vi "Stylus.vi"(9 "Position":T1 {"z (mm)" format="%.1f"; "y (mm)" format="%.1f"; "x (mm)" format="%.1f"}, 10 "Radius":dbl=0.4000000059604645) -> (1 "3D Picture":refnum<vi>(3d-picture), 3 "Scene Object Out":refnum<vi>)   [LabVIEW 2023]
uses:
  <vilib>/picture/3D Picture Control/Object/Create Object (name).vi
  <vilib>/picture/3D Picture Control/Object/Add Object (no reference).vi
  <vilib>/picture/3D Picture Control/NI_3D Picture Control.lvlib
panel:
  out "error out":errorcluster
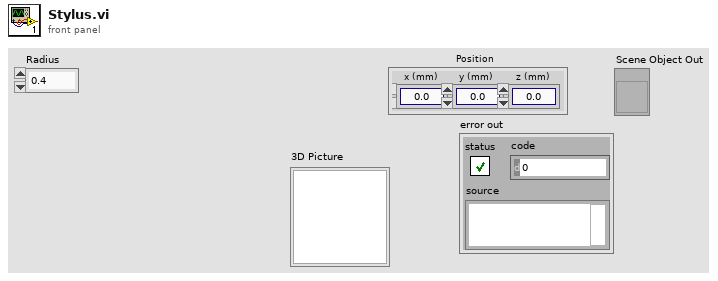
[diagram p1: front panel]
types:
  T1 = cluster{"x (mm)":dbl, "y (mm)":dbl, "z (mm)":dbl}
  T2 = cluster{"Red":sgl, "Green":sgl, "Blue":sgl, "Alpha":sgl}
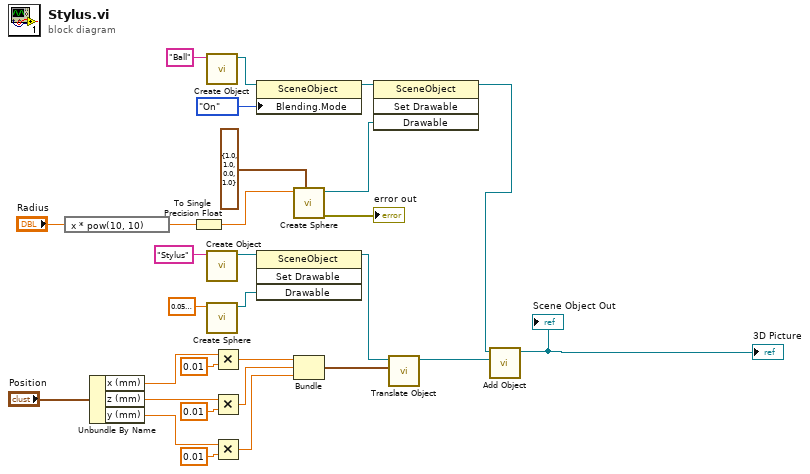
[diagram p0: block diagram]
diagram:
  n1 = expression code="x * pow(10, 10)"("Radius") -> (w9:dbl)
  n2 = Unbundle By Name("Position") -> ("x (mm)"=w19:dbl, "z (mm)"=w18:dbl, "y (mm)"=w17:dbl)
  n3 = To Single Precision Float(number=w9) -> (single precision float=w8:sgl)
  n4 = call-poly <vilib>:"Create Object.vi"("Name"="Ball") -> ("Scene:New Object"=w6:refnum<vi>)  [unwired: 9 in, 1 out]
  n5 = call-poly <vilib>:"Create Object.vi"("Name"="Stylus") -> ("Scene:New Object"=w27:refnum<vi>)  [unwired: 9 in, 1 out]
  n6 = call <vilib>:"Create Sphere.vi"("Radius"=sgl 0.05) -> ("New Sphere Refnum"=w26:refnum<vi>)  [unwired: 9 in, 1 out]
  n7 = Multiply(x=w19, y=0.01) -> (x*y=w16:dbl)
  n8 = Multiply(x=w18, y=0.01) -> (x*y=w24:dbl)
  n9 = Multiply(x=w17, y=0.01) -> (x*y=w15:dbl)
  n10 = property class="SceneObject"(reference=w6, "Blending.Mode"=enum16{"Inherit Value", "Off", "On"}."On" ("Blending:Mode")) -> (reference out=w5:refnum<vi>)  [unwired: 1 in, 1 out]
  n11 = invoke class="SceneObject" method="Set Drawable"(reference=w27, "Drawable"=w26) -> (reference out=w28:refnum<vi>)  [unwired: 2 in, 3 out]
  n12 = call <vilib>:"Create Sphere.vi"("Color"=T2 {"Red"=1.0, "Green"=1.0, "Blue"=0.0, "Alpha"=1.0}, "Radius"=w8) -> ("error out"=→"error out":errorcluster, "New Sphere Refnum"=w12:refnum<vi>)  [unwired: 8 in]
  n13 = Bundle(w16, w24, w15) -> (w22:cluster{dbl, dbl, dbl})  [unwired: 1 in]
  n14 = invoke class="SceneObject" method="Set Drawable"(reference=w5, "Drawable"=w12) -> (reference out=w2:refnum<vi>)  [unwired: 2 in, 3 out]
  n15 = call <vilib>:"Translate Object.vi"("Translation"=w22, "Scene.Object In"=w28) -> ("Scene.Object Out"=w3:refnum<vi>)  [unwired: 8 in, 1 out]
  n16 = call-poly <vilib>:"Add Object.vi"("New Object In"=w3, "Scene Object In"=w2) -> ("Scene Object Out"=→"3D Picture" →"Scene Object Out":refnum<vi>)  [unwired: 8 in, 1 out]
